vi "GetImageFromFile.vi"(8 "error in (no error)":errorcluster, 9 "AddFrame":bool, 10 "Bounds":T2, 11 "path to JPEG file":path) -> (0 "error out":errorcluster, 2 "Image Data":T1, 3 "2D Picture 2":picture)   [LabVIEW 2013]
uses:
  <vilib>/Utility/miscctls.llb/LVBoundsTypeDef.ctl
  <vilib>/picture/picture.llb/imagedata.ctl
  <vilib>/Utility/miscctls.llb/LVPointTypeDef.ctl
panel:
  out "2D Picture":picture
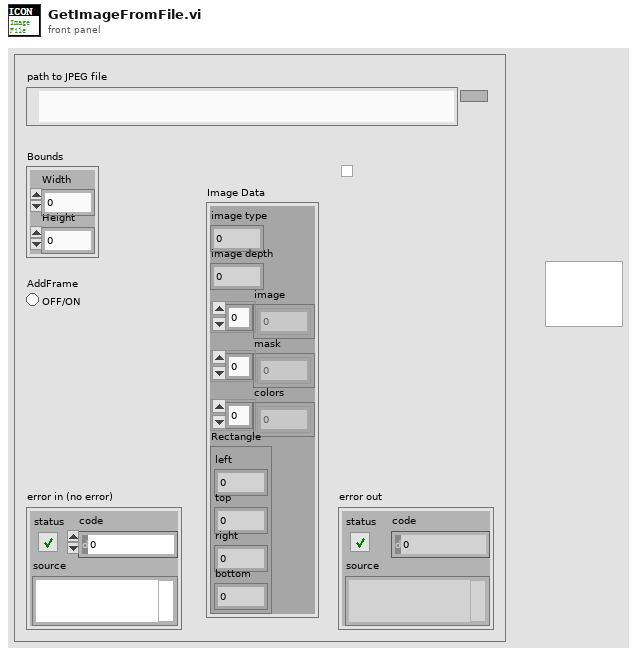
[diagram p1: front panel]
types:
  T1 = typedef "imagedata.ctl" = cluster{"image type":i32, "image depth":i32, "image":u8[], "mask":u8[], "colors":u32[], "Rectangle":cluster{"left":i16, "top":i16, "right":i16, "bottom":i16}}
  T2 = typedef "LVBoundsTypeDef.ctl" = cluster{"Width":u32, "Height":u32}
  T3 = typedef "LVPointTypeDef.ctl" = cluster{"Horizontal":i16, "Vertical":i16}
  T4 = cluster{"Width":i16, "Style":enum32{"Solid", "Dash", "Dot", "DashDot", "DashDotDot"}}
  T5 = cluster{"left":i16, "top":i16, "right":i16, "bottom":i16}
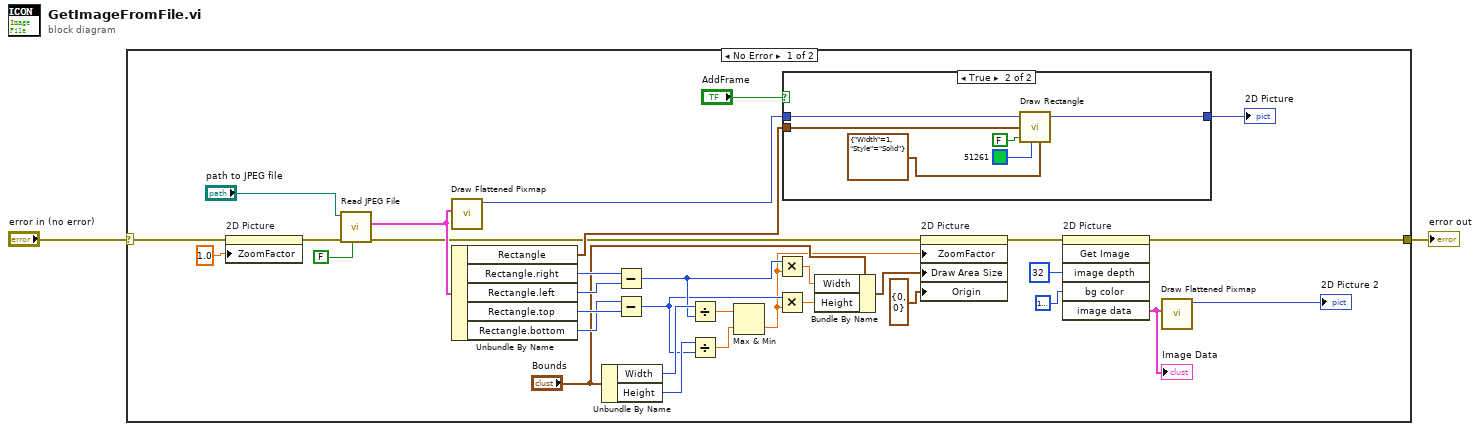
[diagram p0: block diagram]
diagram:
  n1 = case shown="No Error" "error in (no error)" {
    selector: "error in (no error)" -> [w16 w43]
    tunnel: [w10 w43] -> w1
    frame No Error {
      n2 = property on="2D Picture" class="Pict"(error in=w16, "ZoomFactor"=sgl 1.0 ("Zoom Factor 2")) -> (error out=w14:errorcluster)  [unwired: 1 in, 1 out]
      n3 = call <vilib>:"Read JPEG File.vi"("use 8 bit color table"=FALSE, "error in (no error)"=w14, "path to JPEG file"="path to JPEG file") -> ("error out"=w12:errorcluster, "image data"=w32:T1)  [unwired: 6 in, 1 out]
      n4 = call <vilib>:"Draw Flattened Pixmap.vi"("image data"=w32) -> ("new picture"=w17:picture)  [unwired: 8 in]
      n5 = Unbundle By Name(w32) -> ("Rectangle"=w18:T5, "Rectangle.right"=w31:i16, "Rectangle.left"=w30:i16, "Rectangle.top"=w29:i16, "Rectangle.bottom"=w28:i16)
      n6 = Unbundle By Name("Bounds") -> ("Width"=w27:u32, "Height"=w26:u32)
      n7 = Subtract(x=w31, y=w30) -> (x-y=w23:i16)
      n8 = Subtract(x=w28, y=w29) -> (x-y=w22:i16)
      n9 = Divide(x=w27, y=w23) -> (x/y=w24:dbl)
      n10 = Divide(x=w26, y=w22) -> (x/y=w25:dbl)
      n11 = Max & Min(x=w24, y=w25) -> (min(x,y)=w13:dbl)  [unwired: 1 out]
      n12 = Multiply(x=w23, y=w13) -> (x*y=w20:dbl)
      n13 = Multiply(x=w22, y=w13) -> (x*y=w19:dbl)
      n14 = case shown="True" "AddFrame" {
        tunnel: w18 -> [_ w42]
        tunnel: w17 -> [w36 w40]
        tunnel: [w36 w37] -> w5
        frame False {
        }
        frame True {
          n15 = call <vilib>:"Draw Rectangle.vi"("picture"=w40, "rect"=w42, "fill?(F)"=FALSE, "color(black)"=u32 51261, "pen"=T4 {"Width"=1, "Style"=enum."Solid"}) -> ("new picture"=w37:picture)  [unwired: 4 in]
        }
      }
      "2D Picture" <- w5
      n16 = Bundle By Name(cluster="Bounds", "Width"=w20, "Height"=w19) -> (w7:T2)
      n17 = property on="2D Picture" class="Pict"(error in=w12, "ZoomFactor"=w13, "Draw Area Size"=w7, "Origin"=T3 {"Horizontal"=0, "Vertical"=0}) -> (error out=w11:errorcluster)  [unwired: 1 in, 1 out]
      n18 = invoke on="2D Picture" class="Pict" method="Get Image"(error in=w11, "image depth"=32 ("Image Depth"), "bg color"=u32 16777226) -> (error out=w10:errorcluster, "image data"=w8:T1)  [unwired: 3 in, 4 out]
      "Image Data" <- w8
      n19 = call <vilib>:"Draw Flattened Pixmap.vi"("image data"=w8) -> ("new picture"=→"2D Picture 2":picture)  [unwired: 8 in]
    }
    frame Error {
    }
  }
  "error out" <- w1
